vi "Get Path.vi"(0 "Tree Reference In":refnum<vi>, 2 "Child Tag (Current)":string, 5 "error in (no error)":errorcluster) -> (14 "Tree Reference Out":refnum<vi>, 17 "Path":string[](array[string]), 19 "error out":errorcluster)   [LabVIEW 2014]
doc: "Retrieves the parent of the child. Uses the currently selected item if input is left unwired or empty string. Also returns a 1-D array of all members in its family starting at its parent and leading back to its most mature member."
panel:
  # "VI INPUTS"
  # "VI OUTPUTS"
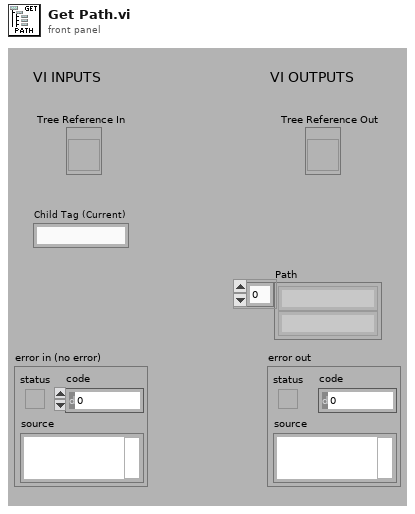
[diagram p1: front panel]
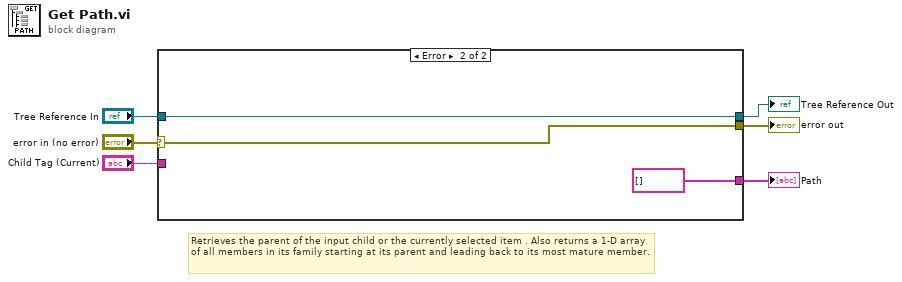
[diagram p0: block diagram]
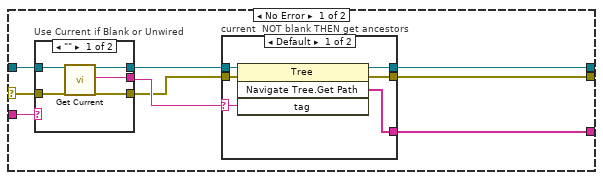
[diagram p2: hidden frame]
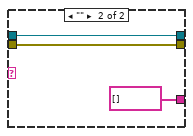
[diagram p4: hidden frame]
diagram:
  # "Retrieves the parent of the input child or the currently selected item . Also returns a 1-D array of all members in its family starting at its parent and leading back to its most mature member."
  n1 = case shown="Error" "error in (no error)" {
    selector: "error in (no error)" -> [w12 w34]
    tunnel: "Tree Reference In" -> [w13 w35]
    tunnel: "Child Tag (Current)" -> [w11 _]
    tunnel: [w15 w35] -> w4
    tunnel: [w7 string[] []] -> w3
    tunnel: [w14 w34] -> w2
    frame No Error {
      n2 = case "Use Current if Blank or Unwired" shown="\"\"" w11 {
        selector: w11 -> [_ w21]
        tunnel: [w19 w23] -> w8
        tunnel: w13 -> [w20 w23]
        tunnel: [w18 w22] -> w9
        tunnel: w12 -> [w17 w22]
        tunnel: [w16 w21] -> w10
        frame "" {
          n3 = call "Get Current.vi"("Tree Reference In"=w20, "error in (no error)"=w17) -> ("Tree Reference Out"=w19:refnum<vi>, "Current Tag"=w16:string, "error out"=w18:errorcluster)  [unwired: 14 in, 1 out]
        }
        frame Default {
        }
      }
      n4 = case "current  NOT blank THEN get ancestors" shown="Default" w10 {
        selector: w10 -> [w24 _]
        tunnel: w8 -> [w29 w32]
        tunnel: [w28 w31] -> w14
        tunnel: [w25 string[] [] ("Navigate Tree:Get Path")] -> w7
        tunnel: [w27 w32] -> w15
        tunnel: w9 -> [w26 w31]
        frame Default {
          n5 = invoke class="Tree" method="Navigate Tree.Get Path"(reference=w29, error in=w26, "tag"=w24) -> (reference out=w27:refnum<vi>, error out=w28:errorcluster, "Navigate Tree:Get Path"=w25:string[])  [unwired: 1 in, 1 out]
        }
        frame "" {
        }
      }
    }
    frame Error {
    }
  }
  "Path" <- w3
  "Tree Reference Out" <- w4
  "error out" <- w2
